vi "Setting Keys.vi"() -> ()   [LabVIEW 2023, in "Manual Cal Standard.lvlib" / "Cal Standard.lvclass"]
uses:
  Cal Standard.lvclass
panel:
  in  "CAL_STD_INFO":string="CalibrationStandardInfo"
  in  "LOAD_FILE_RELATIVE_PATH":string="LoadFileRelativePath"
  in  "SHORT_FILE_RELATIVE_PATH":string="ShortFileRelativePath"
  in  "OPEN_FILE_RELATIVE_PATH":string="OpenFileRelativePath"
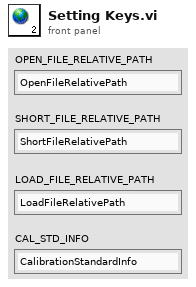
[diagram p1: front panel]
diagram:
